vi "XNET TCP Socket Write (Text).vi"(8 "error in":errorcluster, 9 "timeout ms (25000)":i32=25000, 10 "data":string, 11 "socket in":refnum<k20>) -> (0 "error out":errorcluster, 2 "bytes written":i32, 3 "socket out":refnum<k20>)   [LabVIEW 2018]
doc: "Writes string data to a TCP network connection."
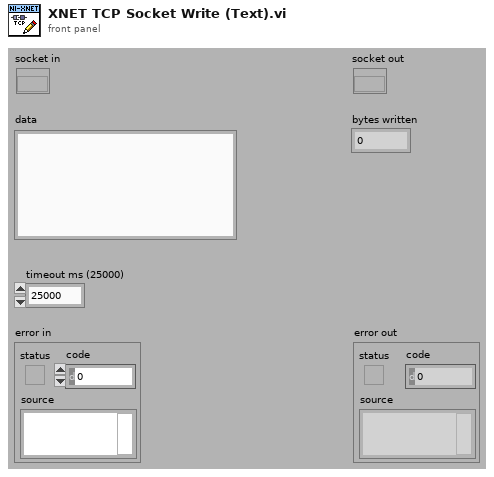
[diagram p1: front panel]
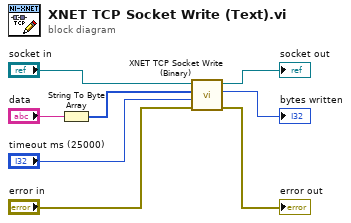
[diagram p0: block diagram]
diagram:
  n1 = String To Byte Array(string="data") -> (unsigned byte array=w6:u8[])
  n2 = call "XNET TCP Socket Write (Binary).vi"("error in"="error in", "timeout ms (25000)"="timeout ms (25000)", "data"=w6, "socket in"="socket in") -> ("error out"=→"error out":errorcluster, "bytes written"=→"bytes written":i32, "socket out"=→"socket out":refnum<k20>)  [unwired: 5 in]
